vi "Koheras_online.vi"(8 "error in":errorcluster, 11 "VISA resource name":refnum<visa-resource-name>="COM3") -> (0 "error out":errorcluster, 2 "Result":cluster{string[], i32[], "Return":string[]}, 3 "VISA resource name out":refnum<visa-resource-name>)   [LabVIEW 2011]
uses:
  Variables/GlobalGetKoherasLaserOnOff.vi
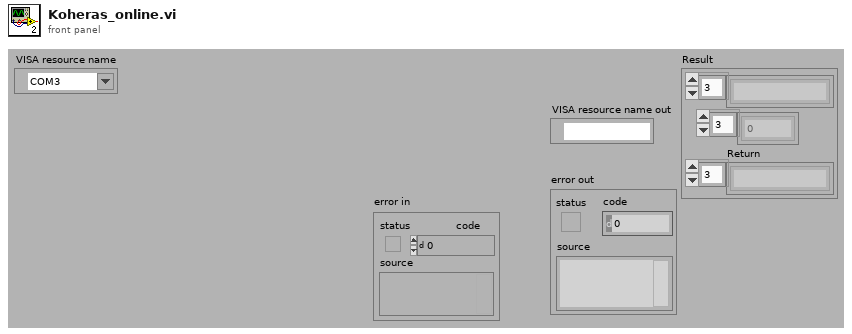
[diagram p1: front panel]
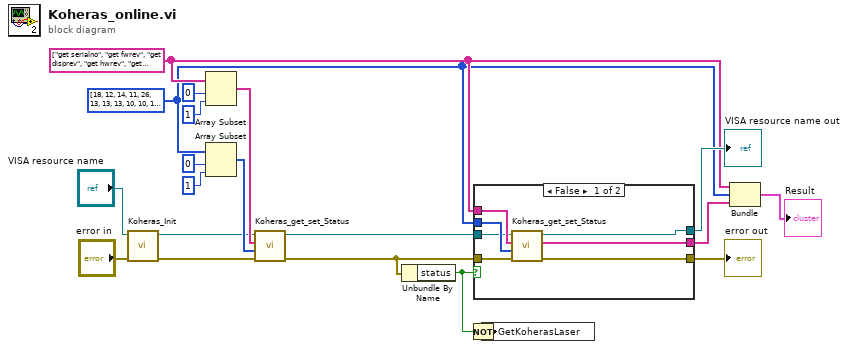
[diagram p0: block diagram]
diagram:
  w5 = i32[] [18, 12, 14, 11, 26, 13, 13, 13, 10, 10, 10, 7, 7, 7, 7, 14, 14, 14, 14, 25, 9, 9, 11]
  w6 = string[] ["get serialno", "get fwrev", "get disprev", "get hwrev", "get almb", "get alm", "get interlock", "get errorcode", "get dcs1", "get dcs2", "get dcs3", "get dc1", "get dc2", "get dc3", "get pd5", "get sensor0", "get sensor1", "get sensor2", "get sensor3", "get datetime", "get state", "get power", "get current"]
  n1 = call "Koheras_Init.vi"("error in"="error in", "VISA resource name"="VISA resource name") -> ("error out"=w10:errorcluster, "VISA resource name out"=w11:refnum<visa-resource-name>)  [unwired: 8 in]
  n2 = Array Subset(array=w6, index=0, length=1) -> (w13:string[])
  n3 = Array Subset(array=w5, index=0, length=1) -> (w12:i32[])
  n4 = call "Koheras_get_set_Status.vi"("error in"=w10, "Array 2"=w12, "Array"=w13, "VISA resource name in"=w11) -> ("error out"=w8:errorcluster, "VISA resource name out"=w9:refnum<visa-resource-name>)  [unwired: 6 out]
  n5 = Unbundle By Name(w8) -> ("status"=w2:bool)
  n6 = Not(x=w2) -> (.not. x?=w1:bool)
  n7 = case shown="False" w2 {
    tunnel: [w27 w28] -> w4
    tunnel: [w26 w30] -> w16
    tunnel: w5 -> [w25 _]
    tunnel: w6 -> [w24 w28]
    tunnel: w9 -> [w23 w29]
    tunnel: w8 -> [w22 w30]
    tunnel: [w21 w29] -> w7
    frame False {
      n8 = call "Koheras_get_set_Status.vi"("error in"=w22, "Array 2"=w25, "Array"=w24, "VISA resource name in"=w23) -> ("error out"=w26:errorcluster, "Return"=w27:string[], "VISA resource name out"=w21:refnum<visa-resource-name>)  [unwired: 5 out]
    }
    frame True {
    }
  }
  "error out" <- w16
  "VISA resource name out" <- w7
  n9 = global write "GlobalGetKoherasLaserOnOff.vi" "GetKoherasLaser"(w1) -> ()
  n10 = Bundle(w6, w5, "Return"=w4) -> (→"Result":cluster{string[], i32[], "Return":string[]})  [unwired: 1 in]
